vi "wait for bytes at serial port.vi"(8 "error in (no error)":errorcluster, 9 "lower limit":i32, 10 "String":string="!", 11 "VISA Refnum in":refnum<visa-resource-name>) -> (0 "error out":errorcluster, 1 "return count":u32, 2 "loop":i32, 3 "VISA Refnum out":refnum<visa-resource-name>)   [LabVIEW 2016]
panel:
  out "Serial Settings:Number of Bytes at Serial Port":u32
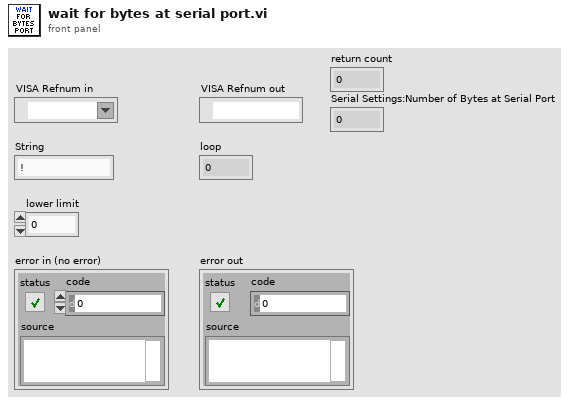
[diagram p1: front panel]
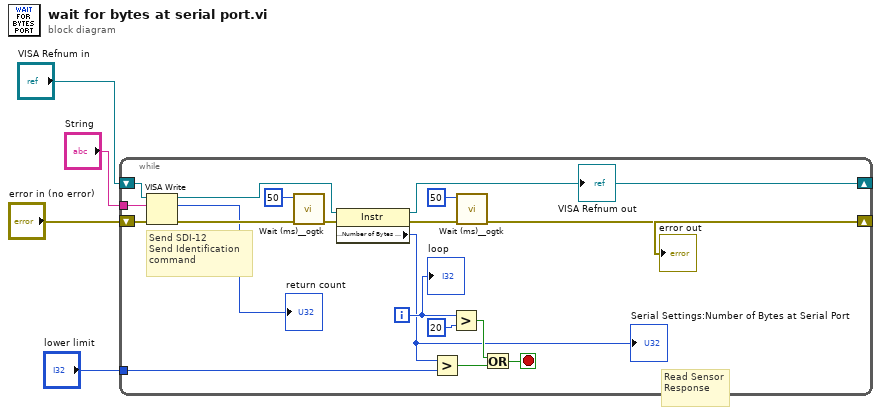
[diagram p0: block diagram]
diagram:
  # "Read Sensor\nResponse"
  n1 = while {
    shift-right: [w13] -> w3
    shift-left: "error in (no error)" -> [w24]
    shift-right: [w22] -> w2
    shift-left: "VISA Refnum in" -> [w10]
    tunnel: "String" -> [w9]
    tunnel: "lower limit" -> [w8]
    i -> [w14]
    stop <- w15 stop-if-true
    # "Send SDI-12 \nSend Identification \ncommand"
    n2 = VISA Write(VISA resource name=w10, write buffer=w9, error in (no error)=w24) -> (VISA resource name out=w23:refnum<visa-resource-name>, return count=→"return count":u32, error out=w25:errorcluster)
    n3 = call "Wait (ms)__ogtk.vi"("error in (no error)"=w25, "milliseconds to wait"=u32 50) -> ("error out"=w19:errorcluster)  [unwired: 8 in, 1 out]
    n4 = property class="Instr"(reference=w23, error in=w19) -> (reference out=w22:refnum<visa-resource-name>, error out=w21:errorcluster, "Serial Settings:Number of Bytes at Serial Port"=w11:u32)
    "Serial Settings:Number of Bytes at Serial Port" <- w11
    n5 = Greater?(x=w11, y=w8) -> (0:w18:bool)
    n6 = Greater?(x=w14, y=20) -> (0:w17:bool)
    n7 = call "Wait (ms)__ogtk.vi"("error in (no error)"=w21, "milliseconds to wait"=u32 50) -> ("error out"=w13:errorcluster)  [unwired: 8 in, 1 out]
    n8 = Or(x=w17, y=w18) -> (x .or. y?=w15:bool)
    "loop" <- w14
  }
  "error out" <- w3
  "VISA Refnum out" <- w2
